vi "FCI_Circle_Blob_Center.vi"(8 "error in (no error)":errorcluster, 10 "Coord ROI":T1 {"Contours"."Type" items=["No Selection", "Point", "Line", "Rectangle", "Oval", "Polygon", "Freehand Region", "Annulus", "Unused2", "Unused3", "Broken Line", "Freehand Line", "Rotated Rectangle"]}, 11 "Image":T2(plugin-control)) -> (0 "error out":errorcluster, 3 "Center Coordinates":cluster{"Center X":dbl, "Center Y":dbl})   [LabVIEW 2019, in "Algorithm.lvclass"]
uses:
  FrameworkOverrides/Algorithm.lvclass
  <vilib>/vision/NI_Vision_Development_Module.lvlib
panel:
  out "Image 2":T2(plugin-control)
  out "X Coord":dbl[](array[numeric])
  out "Array":bool[](array[boolean])
  out "index of element":i32
  out "subarray 2":dbl[](array[numeric])
  out "Number of Particles":i32
  out "Y Coord":dbl[](array[numeric])
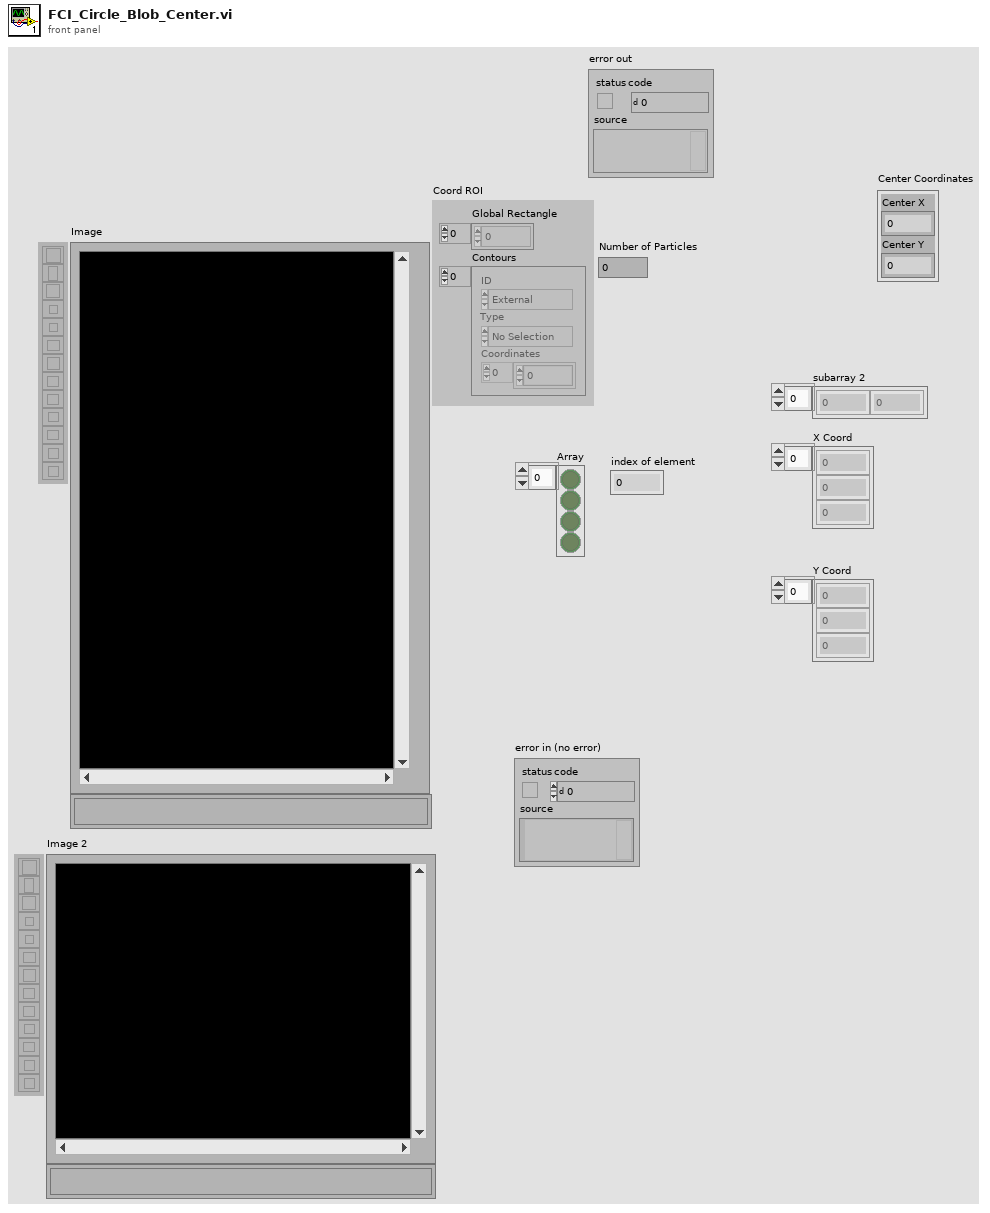
[diagram p1: front panel]
types:
  T1 = typedef "ROI Descriptor" = cluster{"Global Rectangle":i32[], "Contours":cluster{"ID":enum32{"External", "Internal"}, "Type":u32, "Coordinates":i32[]}[]}
  T2 = typedef "IMAQ Image.ctl" = refnum<image>
  T3 = typedef "Particle Parameters" = i32
  T4 = cluster{"Measurement Parameter":T3, "Range Lower Value":dbl, "Range Upper Value":dbl, "Range":bool, "Measurement Type":bool}[]
  T5 = typedef "Image Type" = u32
  T6 = typedef "IMAQ Rectangle" = cluster{"Left":i32, "Top":i32, "Right":i32, "Bottom":i32, "Rotation":dbl}
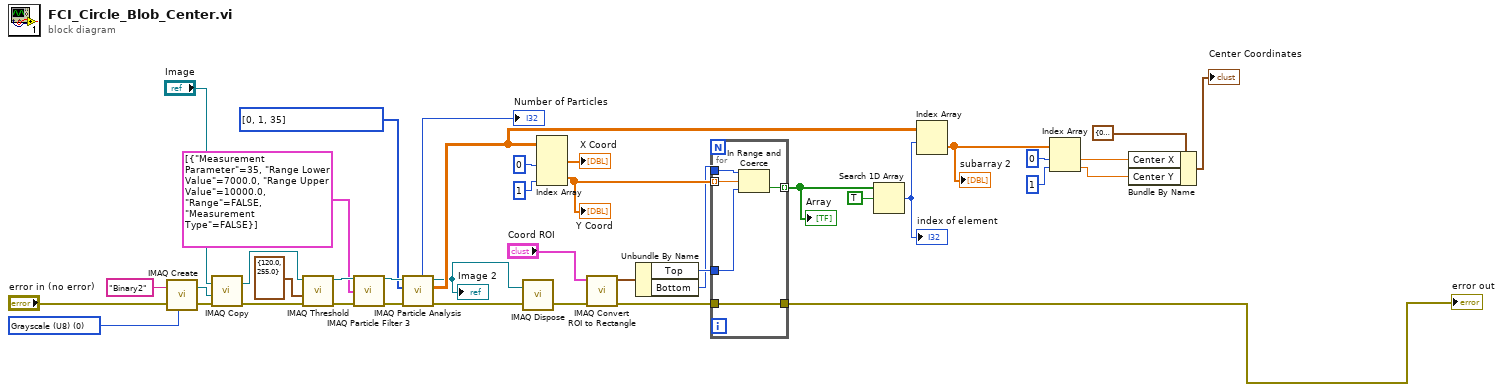
[diagram p0: block diagram]
diagram:
  w32 = T3[] [0, 1, 35] items=["Center of Mass X", "Center of Mass Y", "First Pixel X", "First Pixel Y", "Bounding Rect Left", "Bounding Rect Top", "Bounding Rect Right", "Bounding Rect Bottom", "Max Feret Diameter Start X", "Max Feret Diameter Start Y", "Max Feret Diameter End X", "Max Feret Diameter End Y", "Max Horiz. Segment Length Left", "Max Horiz. Segment Length Right", "Max Horiz. Segment Length Row", "-", "Bounding Rect Width", "Bounding Rect Height", "Bounding Rect Diagonal", "Perimeter", "Convex Hull Perimeter", "Holes' Perimeter", "Max Feret Diameter", "Equivalent Ellipse Major Axis", "Equivalent Ellipse Minor Axis", "Equivalent Ellipse Minor Axis (Feret)", "Equivalent Rect Long Side", "Equivalent Rect Short Side", "Equivalent Rect Diagonal", "Equivalent Rect Short Side (Feret)", "Average Horiz. Segment Length", "Average Vert. Segment Length", "Hydraulic Radius", "Waddel Disk Diameter", "-", "Area", "Holes' Area", "Particle & Holes' Area", "Convex Hull Area", "Image Area", "-", "Number of Holes", "Number of Horiz. Segments", "Number of Vert. Segments", "-", "Orientation", "Max Feret Diameter Orientation", "-", "% Area/Image Area", "% Area/(Particle & Holes' Area)", "Ratio of Equivalent Ellipse Axes", "Ratio of Equivalent Rect Sides", "-", "Elongation Factor", "Compactness Factor", "Heywood Circularity Factor", "Type Factor", "-", "Sum X", "Sum Y", "Sum XX", "Sum XY", "Sum YY", "Sum XXX", "Sum XXY", "Sum XYY", "Sum YYY", "-", "Moment of Inertia XX", "Moment of Inertia XY", "Moment of Inertia YY", "Moment of Inertia XXX", "Moment of Inertia XXY", "Moment of Inertia XYY", "Moment of Inertia YYY", "Norm. Moment of Inertia XX", "Norm. Moment of Inertia XY", "Norm. Moment of Inertia YY", "Norm. Moment of Inertia XXX", "Norm. Moment of Inertia XXY", "Norm. Moment of Inertia XYY", "Norm. Moment of Inertia YYY", "Hu Moment 1", "Hu Moment 2", "Hu Moment 3", "Hu Moment 4", "Hu Moment 5", "Hu Moment 6", "Hu Moment 7"] ("Pixel Measurements")
  w39 = T5 0 items=["Grayscale (U8)", "Grayscale (I16)", "Grayscale (SGL)", "Complex (CSG)", "RGB (U32)", "HSL (U32)", "RGB (U64)", "Grayscale (U16)"] ("Image Type")
  n1 = call "IMAQ Create"("Image Name"="Binary2", "Image Type"=w39, "error in (no error)"="error in (no error)") -> ("New Image"=w38:T2, "error out"=w37:errorcluster)  [unwired: 2 in]
  n2 = call "IMAQ Copy"("error in (no error)"=w37, "Image Dst"=w38, "Image Src"="Image") -> ("error out"=w16:errorcluster, "Image Dst Out"=w31:T2)  [unwired: 3 in]
  n3 = call "IMAQ Threshold"("error in (no error)"=w16, "Range"=cluster{"Lower value":sgl, "Upper value":sgl} {"Lower value"=120.0, "Upper value"=255.0}, "Image Src"=w31) -> ("error out"=w36:errorcluster, "Image Dst Out"=w35:T2)  [unwired: 7 in]
  n4 = call "IMAQ Particle Filter 3"("Image Src"=w35, "Selection Values"=T4 [{"Measurement Parameter"=35, "Range Lower Value"=7000.0, "Range Upper Value"=10000.0, "Range"=FALSE, "Measurement Type"=FALSE}], "error in (no error)"=w36) -> ("Image Dst Out"=w34:T2, "error out"=w33:errorcluster)  [unwired: 10 in, 1 out]
  n5 = call "IMAQ Particle Analysis"("error in (no error)"=w33, "Pixel Measurements"=w32, "Image"=w34) -> ("error out"=w5:errorcluster, "Particle Measurements (Pixels)"=w27:dbl[][], "Image Out (duplicate)"=w3:T2, "Number of Particles"=→"Number of Particles":i32)  [unwired: 3 in, 2 out]
  "Image 2" <- w3
  n6 = call "IMAQ Dispose"("Image"=w3, "error in (no error)"=w5) -> ("error out"=w4:errorcluster)  [unwired: 4 in]
  n7 = Index Array(array=w27, index (col) #1=0 ("disabled index (col)"), index (col) #2=1 ("index (col)")) -> (element #1=→"X Coord":dbl[], element #2=w19:dbl[])  [unwired: 2 in]
  "Y Coord" <- w19
  n8 = call "IMAQ Convert ROI to Rectangle"("error in (no error)"=w4, "ROI Descriptor"="Coord ROI") -> ("error out"=w6:errorcluster, "Rectangle"=w11:T6)  [unwired: 7 in]
  n9 = Unbundle By Name(w11) -> ("Top"=w10:i32, "Bottom"=w9:i32)
  n10 = for {
    tunnel: w19 -> [w45] mode=indexing
    tunnel: [w44] -> w29 mode=indexing
    tunnel: w9 -> [w43]
    tunnel: w10 -> [w42]
    tunnel: w6 -> [w41]
    tunnel: [w41] -> w1
    n11 = In Range and Coerce(upper limit=w43, x=w45, lower limit=w42) -> (In Range?=w44:bool)  [unwired: 1 out]
  }
  "Array" <- w29
  "error out" <- w1
  n12 = Search 1D Array(1D array=w29, element=TRUE) -> (index of element=w26:i32)  [unwired: 1 in]
  "index of element" <- w26
  n13 = Index Array(array=w27, index (row)=w26) -> (element=w25:dbl[])  [unwired: 1 in]
  "subarray 2" <- w25
  n14 = Index Array(array=w25, index #1=0 ("index"), index #2=1 ("index")) -> (element #1=w14:dbl, element #2=w13:dbl)
  n15 = Bundle By Name(cluster=cluster{"Center X":dbl, "Center Y":dbl} {"Center X"=0.0, "Center Y"=0.0}, "Center X"=w14, "Center Y"=w13) -> (→"Center Coordinates":cluster{"Center X":dbl, "Center Y":dbl})
